vi "Generate Map.vi"(5 "Elevation Angle":i32, 7 "3d Points":cluster{"Data":sgl, "Data":sgl, "Data":sgl}[](array[cluster]), 8 "Sensor Yaw angle (rad)":sgl, 9 "Depth scalar":dbl, 10 "Sensor position":cluster{"X":sgl, "Y":sgl, "Z":sgl}, 11 "Chunks in":T1(array[cluster])) -> (3 "Chunks out":T1(array[cluster]))   [LabVIEW 2014]
uses:
  <vilib>/Analysis/coordinate.llb/2D Cartesian Coordinate Rotation (Scalar).vi
  <vilib>/Analysis/NI_AALPro.lvlib
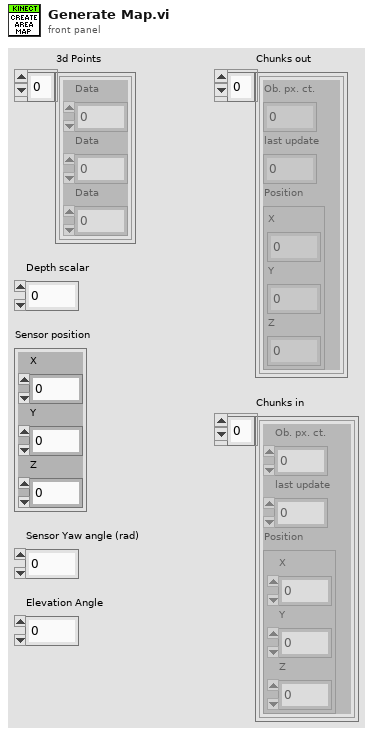
[diagram p1: front panel]
types:
  T1 = cluster{"Ob. px. ct.":u8, "last update":u32, "Position":cluster{"X":i32, "Y":i32, "Z":i32}}[]
  T2 = cluster{"Ob. px. ct.":u8, "last update":u32, "Position":cluster{"X":i32, "Y":i32, "Z":i32}}
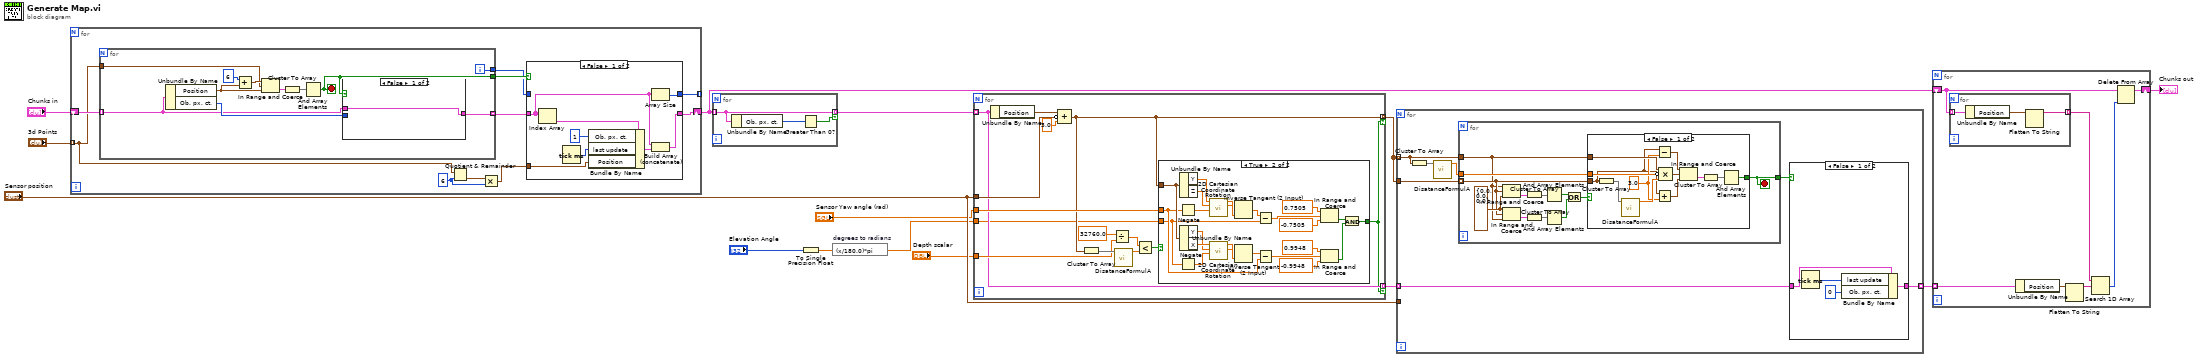
[diagram p0: block diagram]
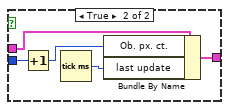
[diagram p6: hidden frame]
diagram:
  n1 = for {
    tunnel: "3d Points" -> [w17] mode=indexing
    shift-right: [w21] -> w2
    shift-left: "Chunks in" -> [w24]
    tunnel: [w19] -> _ mode=indexing
    w15 = 6 ("y")
    n2 = for {
      tunnel: w24 -> [w38] mode=indexing
      tunnel: w17 -> [w42]
      tunnel: [w37] -> w22 mode=indexing
      tunnel: [w36] -> w23
      tunnel: [w35] -> w20
      i -> [w35]
      stop <- w36 stop-if-true
      n3 = Unbundle By Name(w38) -> ("Position"=w43:cluster{"X":i32, "Y":i32, "Z":i32}, "Ob. px. ct."=w39:u8)
      n4 = Add(x=6, y=w43) -> (x+y=w44:cluster{"X":i32, "Y":i32, "Z":i32})
      n5 = In Range and Coerce(upper limit=w44, x=w42, lower limit=w43) -> (In Range?=w41:cluster{"Data":bool, "Data":bool, "Data":bool})  [unwired: 1 out]
      n6 = Cluster To Array(cluster=w41) -> (array=w40:bool[])
      n7 = And Array Elements(Boolean array=w40) -> (logical AND=w36:bool)
      n8 = case shown="False" w36 {
        tunnel: w39 -> [_ w51]
        tunnel: w38 -> [w46 w50]
        tunnel: [w46 w48] -> w37
        frame False {
        }
        frame True {
          n9 = Increment(x=w51) -> (x+1=w49:u8)
          n10 = Tick Count (ms)() -> (millisecond timer value=w47:u32)
          n11 = Bundle By Name(cluster=w50, "Ob. px. ct."=w49, "last update"=w47) -> (w48:T2)
        }
      }
    }
    n12 = Quotient & Remainder(x=w17, y=w15) -> (floor(x/y)=w16:cluster{"Data":sgl, "Data":sgl, "Data":sgl})  [unwired: 1 out]
    n13 = Multiply(x=w16, y=w15) -> (x*y=w18:cluster{"Data":sgl, "Data":sgl, "Data":sgl})
    n14 = case shown="False" w23 {
      tunnel: w18 -> [w30 _]
      tunnel: w22 -> [w27 w34]
      tunnel: [w29 w34] -> w21
      tunnel: w20 -> [_ w33]
      tunnel: [w28 w33] -> w19
      frame False {
        n15 = Index Array(array=w27) -> (element=w26:T2)  [unwired: 1 in]
        n16 = Tick Count (ms)() -> (millisecond timer value=w25:u32)
        n17 = Bundle By Name(cluster=w26, "Ob. px. ct."=u8 1, "last update"=w25, "Position"=w30) -> (w32:T2)
        n18 = Array Size(array=w27) -> (size(s)=w28:i32)
        n19 = Build Array (concatenate)(w27, w32) -> (w29:T1)
      }
      frame True {
      }
    }
  }
  n20 = for {
    tunnel: w2 -> [w53] mode=indexing
    tunnel: [w53] -> w10 mode=indexing if=w52
    n21 = Unbundle By Name(w53) -> ("Ob. px. ct."=w54:u8)
    n22 = Greater Than 0?(x=w54) -> (x > 0?=w52:bool)
  }
  n23 = To Single Precision Float(number="Elevation Angle") -> (single precision float=w6:sgl)
  n24 = expression code="(x/180.0)*pi" "degrees to radians"(w6) -> (w4:sgl)
  n25 = for {
    tunnel: "Sensor position" -> [w67]
    tunnel: "Sensor Yaw angle (rad)" -> [w65]
    tunnel: w10 -> [w58] mode=indexing
    tunnel: w4 -> [w55]
    tunnel: "Depth scalar" -> [w63]
    tunnel: [w58] -> w14 mode=indexing if=w56
    tunnel: [w57] -> w13 mode=indexing if=w56
    n26 = Unbundle By Name(w58) -> ("Position"=w68:cluster{"X":i32, "Y":i32, "Z":i32})
    n27 = Compound Arithmetic op=unknown(w68, invert w67, sgl 3.0) -> (w57:cluster{"X":sgl, "Y":sgl, "Z":sgl})
    n28 = Cluster To Array(cluster=w57) -> (array=w64:sgl[])
    n29 = Divide(x=32760.0, y=w63) -> (x/y=w60:dbl)
    n30 = call "DisatanceFormulA.vi"("A"=w64) -> ("Distance"=w61:dbl)  [unwired: 10 in]
    n31 = Less?(x=w60, y=w61) -> (x < y?=w59:bool)
    n32 = case shown="True" w59 {
      tunnel: w57 -> [_ w88]
      tunnel: w65 -> [_ w87]
      tunnel: [_ w77] -> w56
      tunnel: w55 -> [_ w69]
      frame False {
      }
      frame True {
        n33 = Unbundle By Name(w88) -> ("Y"=w86:sgl, "Z"=w85:sgl)
        n34 = Negate(x=w87) -> (-x=w84:sgl)
        n35 = Unbundle By Name(w88) -> ("Y"=w74:sgl, "X"=w75:sgl)
        n36 = Negate(x=w69) -> (-x=w76:sgl)
        n37 = call-poly <vilib>:"2D Cartesian Coordinate Rotation.vi"("theta"=w84, "y"=w85, "x"=w86) -> ("y out"=w82:dbl, "x out"=w83:dbl)  [unwired: 6 in, 1 out]
        n38 = call-poly <vilib>:"2D Cartesian Coordinate Rotation.vi"("theta"=w76, "y"=w74, "x"=w75) -> ("y out"=w72:dbl, "x out"=w73:dbl)  [unwired: 6 in, 1 out]
        n39 = Inverse Tangent (2 Input)(1:w83, 2:w82) -> (0:w71:dbl)
        n40 = Inverse Tangent (2 Input)(1:w73, 2:w72) -> (0:w92:dbl)
        n41 = Subtract(x=w71, y=w69) -> (x-y=w70:dbl)
        n42 = Subtract(x=w92, y=w87) -> (x-y=w89:dbl)
        n43 = In Range and Coerce(upper limit=0.7505, x=w70, lower limit=-0.7505 ("upper limit")) -> (In Range?=w79:bool)  [unwired: 1 out]
        n44 = In Range and Coerce(upper limit=0.9948, x=w89, lower limit=-0.9948) -> (In Range?=w78:bool)  [unwired: 1 out]
        n45 = And(x=w79, y=w78) -> (x .and. y?=w77:bool)
      }
    }
  }
  n46 = for {
    tunnel: w13 -> [w98] mode=indexing
    tunnel: "Sensor position" -> [_]
    tunnel: w13 -> [w99]
    tunnel: w14 -> [w94] mode=indexing
    tunnel: [w93] -> w3 mode=indexing
    n47 = Cluster To Array(cluster=w98) -> (array=w97:sgl[])
    n48 = call "DisatanceFormulA.vi"("A"=w97) -> ("Distance"=w96:dbl)  [unwired: 10 in]
    n49 = for {
      tunnel: w99 -> [w108] mode=indexing
      tunnel: w98 -> [w106]
      tunnel: w96 -> [w107]
      tunnel: [w105] -> w95
      stop <- w105 stop-if-true
      w114 = cluster{"X":sgl, "Y":sgl, "Z":sgl} {"X"=0.0, "Y"=0.0, "Z"=0.0} ("lower limit")
      n50 = In Range and Coerce(upper limit=w106, x=w108, lower limit=w114) -> (In Range?=w116:cluster{"X":bool, "Y":bool, "Z":bool})  [unwired: 1 out]
      n51 = In Range and Coerce(upper limit=w114, x=w108, lower limit=w106) -> (In Range?=w112:cluster{"X":bool, "Y":bool, "Z":bool})  [unwired: 1 out]
      n52 = Cluster To Array(cluster=w116) -> (array=w115:bool[])
      n53 = Cluster To Array(cluster=w112) -> (array=w113:bool[])
      n54 = And Array Elements(Boolean array=w115) -> (logical AND=w111:bool)
      n55 = And Array Elements(Boolean array=w113) -> (logical AND=w110:bool)
      n56 = Or(x=w111, y=w110) -> (x .or. y?=w109:bool)
      n57 = case shown="False" w109 {
        tunnel: w108 -> [w121 _]
        tunnel: w107 -> [w127 _]
        tunnel: w106 -> [w125 _]
        tunnel: [w117 _] -> w105
        frame False {
          w123 = 3.0 ("y")
          n58 = Cluster To Array(cluster=w121) -> (array=w128:sgl[])
          n59 = call "DisatanceFormulA.vi"("A"=w128) -> ("Distance"=w126:dbl)  [unwired: 10 in]
          n60 = Subtract(x=w121, y=w123) -> (x-y=w124:cluster{"X":dbl, "Y":dbl, "Z":dbl})
          n61 = Add(x=w121, y=w123) -> (x+y=w122:cluster{"X":dbl, "Y":dbl, "Z":dbl})
          n62 = Compound Arithmetic op=MULTIPLY(w125, invert w127, w126) -> (w120:cluster{"X":dbl, "Y":dbl, "Z":dbl})
          n63 = In Range and Coerce(upper limit=w124, x=w120, lower limit=w122) -> (In Range?=w119:cluster{"X":bool, "Y":bool, "Z":bool})  [unwired: 1 out]
          n64 = Cluster To Array(cluster=w119) -> (array=w118:bool[])
          n65 = And Array Elements(Boolean array=w118) -> (logical AND=w117:bool)
        }
        frame True {
        }
      }
    }
    n66 = case shown="False" w95 {
      tunnel: w94 -> [w103 w104]
      tunnel: [w100 w104] -> w93
      frame False {
        n67 = Tick Count (ms)() -> (millisecond timer value=w101:u32)
        n68 = Bundle By Name(cluster=w103, "last update"=w101, "Ob. px. ct."=u8 0) -> (w100:T2)
      }
      frame True {
      }
    }
  }
  n69 = for {
    tunnel: w3 -> [w135] mode=indexing
    shift-right: [w129] -> w1
    shift-left: w2 -> [w130]
    n70 = for {
      tunnel: w130 -> [w138] mode=indexing
      tunnel: [w136] -> w133 mode=indexing
      n71 = Unbundle By Name(w138) -> ("Position"=w137:cluster{"X":i32, "Y":i32, "Z":i32})
      n72 = Flatten To String(anything=w137) -> (data string=w136:string)  [unwired: 3 in, 2 out]
    }
    n73 = Unbundle By Name(w135) -> ("Position"=w134:cluster{"X":i32, "Y":i32, "Z":i32})
    n74 = Flatten To String(anything=w134) -> (data string=w132:string)  [unwired: 3 in, 2 out]
    n75 = Search 1D Array(1D array=w133, element=w132) -> (index of element=w131:i32)  [unwired: 1 in]
    n76 = Delete From Array(array=w130, index=w131) -> (array with subset deleted=w129:T1)  [unwired: 1 in, 1 out]
  }
  "Chunks out" <- w1
